vi "Set #Cubes.vi"(8 "error in (no error)":errorcluster, 11 "CCDCamera in":refnum<class "CCDCamera.lvclass">) -> (0 "error out":errorcluster, 3 "CCDCamera out":refnum<class "CCDCamera.lvclass">)   [LabVIEW 2018, in "CCDCamera.lvclass"]
uses:
  CCDCamera.lvclass
  C:/Users/observer/Desktop/SPARC4_ACS/SPARC4_ACS/Simulated_CCD_Camera/Simulated_CCD_Camera.lvclass
  Simulated_CCD_Camera/Simulated_CCD_Camera.lvclass/Simulated_CCD_Camera.ctl
  Interface/Interface.lvclass/Interface.ctl
  Interface/Interface.lvclass
  Simulated_CCD_Camera/Simulated_CCD_Camera.lvclass
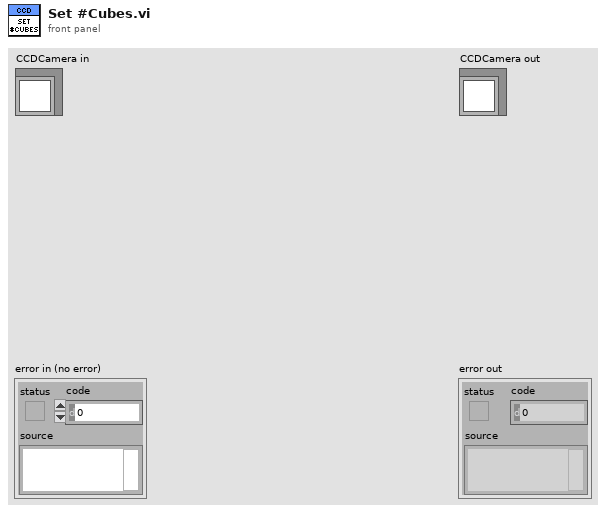
[diagram p1: front panel]
types:
  T1 = cluster{"COOLER_POWER_STATUS":u16, "TEMP":i32, "EXPTIME":dbl, "#FRAMES":u32, "#CUBES":u32}
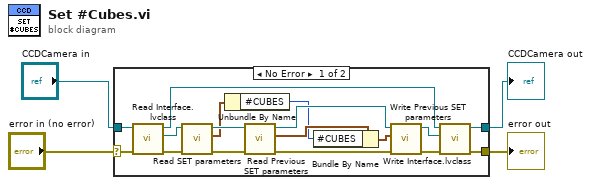
[diagram p0: block diagram]
diagram:
  n1 = case shown="No Error" "error in (no error)" {
    selector: "error in (no error)" -> [w20 w23]
    tunnel: [w19 w23] -> w3
    tunnel: [w18 w22] -> w1
    tunnel: "CCDCamera in" -> [w21 w22]
    frame No Error {
      n2 = call "Read Interface.lvclass.vi"("error in (no error)"=w20, "Simulated_CCD_Camera in"=w21) -> ("error out"=w9:errorcluster, "Interface.lvclass"=w10:refnum<class "Interface.lvclass">, "Simulated_CCD_Camera out"=w17:refnum<class "CCDCamera.lvclass">)  [unwired: 7 in]
      n3 = call "Read SET parameters.vi"("error in (no error)"=w9, "Interface in"=w10) -> ("error out"=w8:errorcluster, "SET parameters"=w6:T1, "Interface out"=w7:refnum<class "Interface.lvclass">)  [unwired: 7 in]
      n4 = Unbundle By Name(w6) -> ("#CUBES"=w5:u32)
      n5 = call "Read Previous SET parameters.vi"("error in (no error)"=w8, "Interface in"=w7) -> ("error out"=w14:errorcluster, "Previous SET parameters"=w16:T1, "Interface out"=w13:refnum<class "Interface.lvclass">)  [unwired: 7 in]
      n6 = Bundle By Name(cluster=w16, "#CUBES"=w5) -> (w15:T1)
      n7 = call "Write Previous SET parameters.vi"("error in (no error)"=w14, "Previous SET parameters"=w15, "Interface in"=w13) -> ("error out"=w12:errorcluster, "Interface out"=w11:refnum<class "Interface.lvclass">)  [unwired: 7 in]
      n8 = call "Write Interface.lvclass.vi"("error in (no error)"=w12, "Interface.lvclass"=w11, "Simulated_CCD_Camera in"=w17) -> ("error out"=w19:errorcluster, "Simulated_CCD_Camera out"=w18:refnum<class "CCDCamera.lvclass">)  [unwired: 7 in]
    }
    frame Error {
    }
  }
  "error out" <- w3
  "CCDCamera out" <- w1
